vi "PROXY_create_queues.vi"(8 "error_in":errorcluster, 11 "all_config_info_in":T1) -> (0 "error_out":errorcluster, 3 "all_config_info_out":T1)   [LabVIEW 2020]
uses:
  ini/typedef/PROXY_all_config_info.ctl
  ini/typedef/PROXY_main_ini_file.ctl
  typedef/PROXY_queue_refnums.ctl
  typedef/STATION_queue_element.ctl
  STATION/ST_SQL_sequence_state.ctl
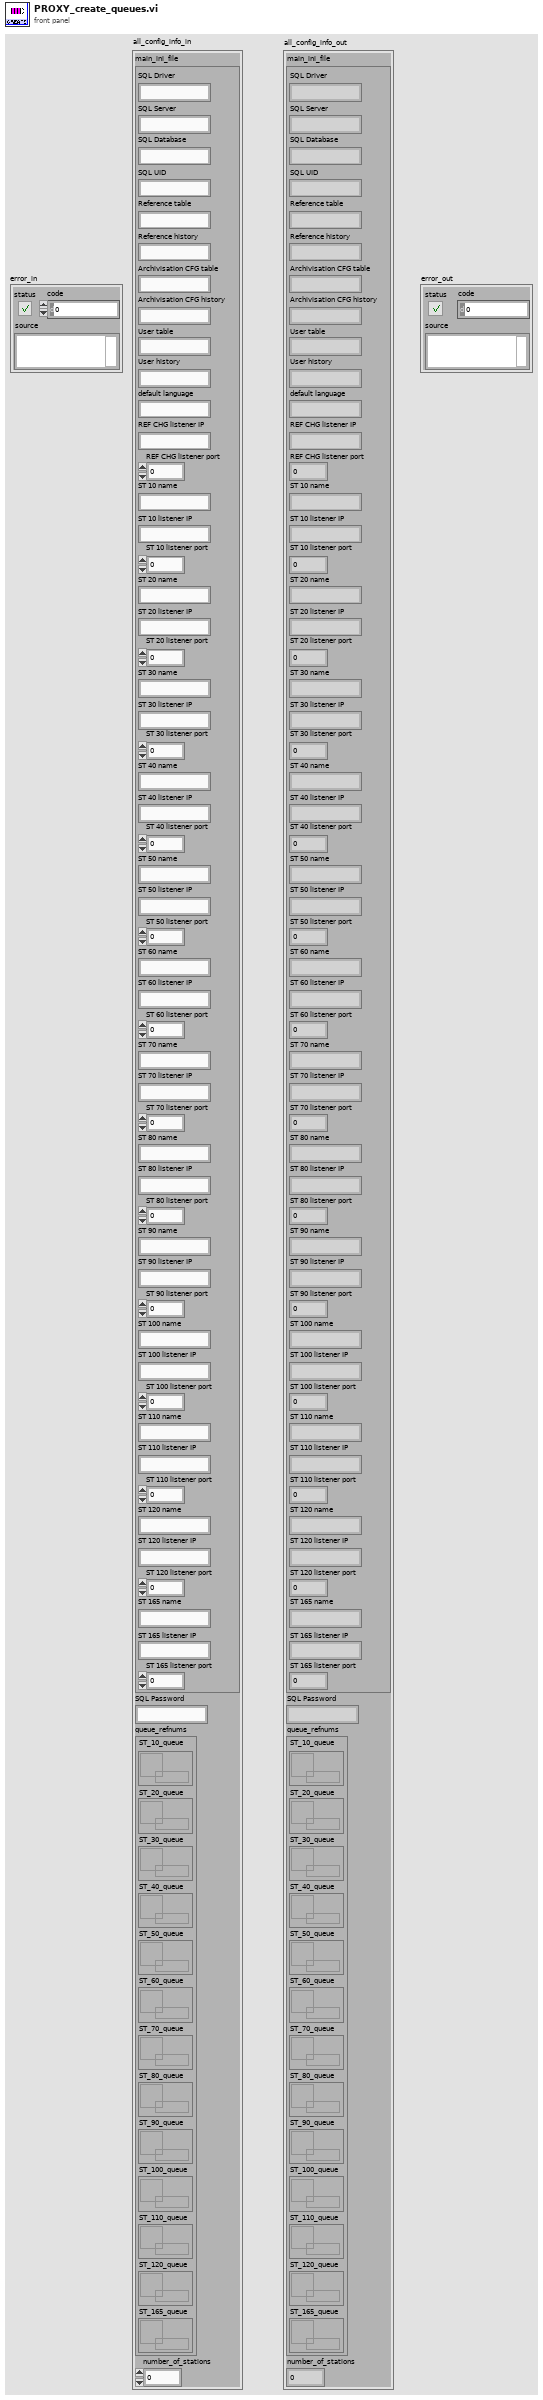
[diagram p1: front panel]
types:
  T1 = typedef "PROXY_all_config_info.ctl" = cluster{"main_ini_file":T2, "SQL Password":string, "queue_refnums":T3, "number_of_stations":i32}
  T2 = typedef "PROXY_main_ini_file.ctl" = cluster{"SQL Driver":string, "SQL Server":string, "SQL Database":string, "SQL UID":string, "Reference table":string, "Reference history":string, "Archivisation CFG table":string, "Archivisation CFG history":string, "User table":string, "User history":string, "default language":string, "REF CHG listener IP":string, "REF CHG listener port":u16, "ST 10 name":string, "ST 10 listener IP":string, "ST 10 listener port":u16, "ST 20 name":string, "ST 20 listener IP":string, "ST 20 listener port":u16, "ST 30 name":string, "ST 30 listener IP":string, "ST 30 listener port":u16, "ST 40 name":string, "ST 40 listener IP":string, "ST 40 listener port":u16, "ST 50 name":string, "ST 50 listener IP":string, "ST 50 listener port":u16, "ST 60 name":string, "ST 60 listener IP":string, "ST 60 listener port":u16, "ST 70 name":string, "ST 70 listener IP":string, "ST 70 listener port":u16, "ST 80 name":string, "ST 80 listener IP":string, "ST 80 listener port":u16, "ST 90 name":string, "ST 90 listener IP":string, "ST 90 listener port":u16, "ST 100 name":string, "ST 100 listener IP":string, "ST 100 listener port":u16, "ST 110 name":string, "ST 110 listener IP":string, "ST 110 listener port":u16, "ST 120 name":string, "ST 120 listener IP":string, "ST 120 listener port":u16, "ST 165 name":string, "ST 165 listener IP":string, "ST 165 listener port":u16}
  T3 = typedef "PROXY_queue_refnums.ctl" = cluster{"ST_10_queue":refnum<queue>, "ST_20_queue":refnum<queue>, "ST_30_queue":refnum<queue>, "ST_40_queue":refnum<queue>, "ST_50_queue":refnum<queue>, "ST_60_queue":refnum<queue>, "ST_70_queue":refnum<queue>, "ST_80_queue":refnum<queue>, "ST_90_queue":refnum<queue>, "ST_100_queue":refnum<queue>, "ST_110_queue":refnum<queue>, "ST_120_queue":refnum<queue>, "ST_165_queue":refnum<queue>}
  T4 = typedef "STATION_queue_element.ctl" = cluster{"state":T5, "variable":variant}
  T5 = typedef "ST_SQL_sequence_state.ctl" = enum16{"initialize", "get_next_state", "send_to_SQL", "send_to_PLC", "error", "stop"}
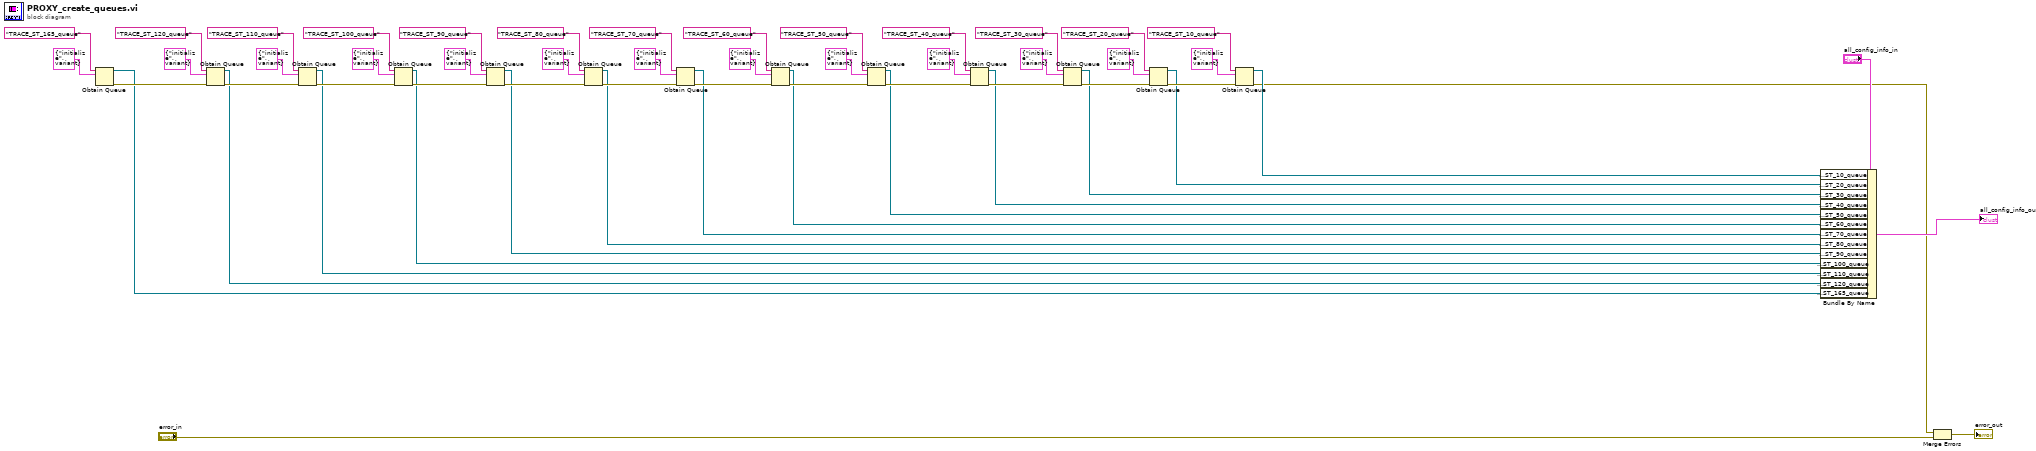
[diagram p0: block diagram]
diagram:
  n1 = Obtain Queue(name (unnamed)="TRACE_ST_165_queue", element data type=T4 {"state"=enum."initialize", "variable"=variant} ("STATION_queue_element")) -> (queue out=w2:refnum<queue>, error out=w3:errorcluster)  [unwired: 3 in, 1 out]
  n2 = Obtain Queue(name (unnamed)="TRACE_ST_120_queue", element data type=T4 {"state"=enum."initialize", "variable"=variant} ("STATION_queue_element"), error in (no error)=w3) -> (queue out=w6:refnum<queue>, error out=w15:errorcluster)  [unwired: 2 in, 1 out]
  n3 = Obtain Queue(name (unnamed)="TRACE_ST_110_queue", element data type=T4 {"state"=enum."initialize", "variable"=variant} ("STATION_queue_element"), error in (no error)=w15) -> (queue out=w7:refnum<queue>, error out=w16:errorcluster)  [unwired: 2 in, 1 out]
  n4 = Obtain Queue(name (unnamed)="TRACE_ST_100_queue", element data type=T4 {"state"=enum."initialize", "variable"=variant} ("STATION_queue_element"), error in (no error)=w16) -> (queue out=w8:refnum<queue>, error out=w17:errorcluster)  [unwired: 2 in, 1 out]
  n5 = Obtain Queue(name (unnamed)="TRACE_ST_90_queue", element data type=T4 {"state"=enum."initialize", "variable"=variant} ("STATION_queue_element"), error in (no error)=w17) -> (queue out=w9:refnum<queue>, error out=w18:errorcluster)  [unwired: 2 in, 1 out]
  n6 = Obtain Queue(name (unnamed)="TRACE_ST_80_queue", element data type=T4 {"state"=enum."initialize", "variable"=variant} ("STATION_queue_element"), error in (no error)=w18) -> (queue out=w10:refnum<queue>, error out=w19:errorcluster)  [unwired: 2 in, 1 out]
  n7 = Obtain Queue(name (unnamed)="TRACE_ST_70_queue", element data type=T4 {"state"=enum."initialize", "variable"=variant} ("STATION_queue_element"), error in (no error)=w19) -> (queue out=w11:refnum<queue>, error out=w20:errorcluster)  [unwired: 2 in, 1 out]
  n8 = Obtain Queue(name (unnamed)="TRACE_ST_60_queue", element data type=T4 {"state"=enum."initialize", "variable"=variant} ("STATION_queue_element"), error in (no error)=w20) -> (queue out=w12:refnum<queue>, error out=w21:errorcluster)  [unwired: 2 in, 1 out]
  n9 = Obtain Queue(name (unnamed)="TRACE_ST_50_queue", element data type=T4 {"state"=enum."initialize", "variable"=variant} ("STATION_queue_element"), error in (no error)=w21) -> (queue out=w13:refnum<queue>, error out=w22:errorcluster)  [unwired: 2 in, 1 out]
  n10 = Obtain Queue(name (unnamed)="TRACE_ST_40_queue", element data type=T4 {"state"=enum."initialize", "variable"=variant} ("STATION_queue_element"), error in (no error)=w22) -> (queue out=w14:refnum<queue>, error out=w23:errorcluster)  [unwired: 2 in, 1 out]
  n11 = Obtain Queue(name (unnamed)="TRACE_ST_30_queue", element data type=T4 {"state"=enum."initialize", "variable"=variant} ("STATION_queue_element"), error in (no error)=w23) -> (queue out=w48:refnum<queue>, error out=w51:errorcluster)  [unwired: 2 in, 1 out]
  n12 = Obtain Queue(name (unnamed)="TRACE_ST_20_queue", element data type=T4 {"state"=enum."initialize", "variable"=variant} ("STATION_queue_element"), error in (no error)=w51) -> (queue out=w49:refnum<queue>, error out=w50:errorcluster)  [unwired: 2 in, 1 out]
  n13 = Obtain Queue(name (unnamed)="TRACE_ST_10_queue", element data type=T4 {"state"=enum."initialize", "variable"=variant} ("STATION_queue_element"), error in (no error)=w50) -> (queue out=w54:refnum<queue>, error out=w1:errorcluster)  [unwired: 2 in, 1 out]
  n14 = Bundle By Name(cluster="all_config_info_in", "queue_refnums.ST_10_queue"=w54, "queue_refnums.ST_20_queue"=w49, "queue_refnums.ST_30_queue"=w48, "queue_refnums.ST_40_queue"=w14, "queue_refnums.ST_50_queue"=w13, "queue_refnums.ST_60_queue"=w12, "queue_refnums.ST_70_queue"=w11, "queue_refnums.ST_80_queue"=w10, "queue_refnums.ST_90_queue"=w9, "queue_refnums.ST_100_queue"=w8, "queue_refnums.ST_110_queue"=w7, "queue_refnums.ST_120_queue"=w6, "queue_refnums.ST_165_queue"=w2) -> (→"all_config_info_out":T1)
  n15 = Merge Errors(w1, "error_in") -> (→"error_out":errorcluster)
